vi "replace_bytes_in_type_descriptor.vi"(9 "offset (-1: current position)":i32=-1, 10 "value to write":refnum<class "Bytes.lvclass">, 11 "LVData in":refnum<class "variant.lvclass">) -> (3 "LVData out":refnum<class "variant.lvclass">)   [LabVIEW 2020, in "variant.lvlib" / "variant.lvclass"]
uses:
  variant.lvclass
  Bytes/Bytes.lvclass
  variant.lvclass/variant.ctl
  Bytes/Bytes.lvclass/Bytes.ctl
  Bytes/to_data.vi
  Type Descriptor/TD.lvclass
  C:/projects/OpenG-Variant-Data-Library/source/library/Bytes/Bytes.lvclass
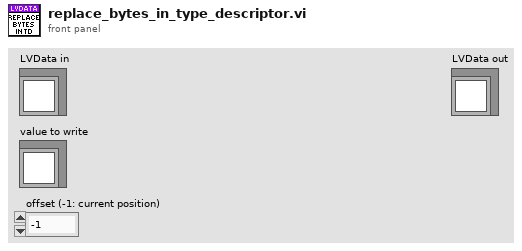
[diagram p1: front panel]
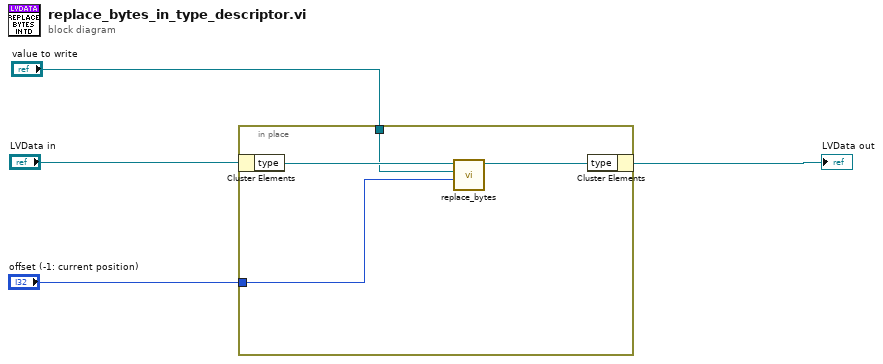
[diagram p0: block diagram]
diagram:
  n1 = in-place {
    in-place-border: "offset (-1: current position)" -> [w7]
    in-place-border: "value to write" -> [w5]
    n2 = in-place-cluster #1("LVData in") -> ("type"=w8:refnum<class "TD.lvclass">)
    n3 = call "replace_bytes.vi"("offset (-1: current position)"=w7, "bytes to write"=w5, "Bytes in"=w8) -> ("Bytes out"=w6:refnum<class "TD.lvclass">)  [unwired: 8 in]
    n4 = in-place-cluster #1("type"=w6) -> (→"LVData out":refnum<class "variant.lvclass">)
  }
